vi "get_user_details.vi"(11 "error in (no error)":errorcluster) -> (4 "Name 2":string caption="Enter your name", 6 "Birthday 2":timestamp caption="Select Birthday" format="%<%x>T", 8 "Back_out":T1 caption="Back", 10 "path":path, 15 "error out":errorcluster)   [LabVIEW 2023]
doc: "get the user details."
uses:
  custom_elements/continue.ctl
  custom_elements/back_button.ctl
  <vilib>/Utility/error.llb/Trim Whitespace One-Sided.vi
panel:
  in  "Back":T1
  in  "stop":T2
  in  "Name":string caption="The Name Bestowed Upon Thee"
  in  "Birthday":timestamp caption="The Day of Thy First Light" format="%<%x>T"
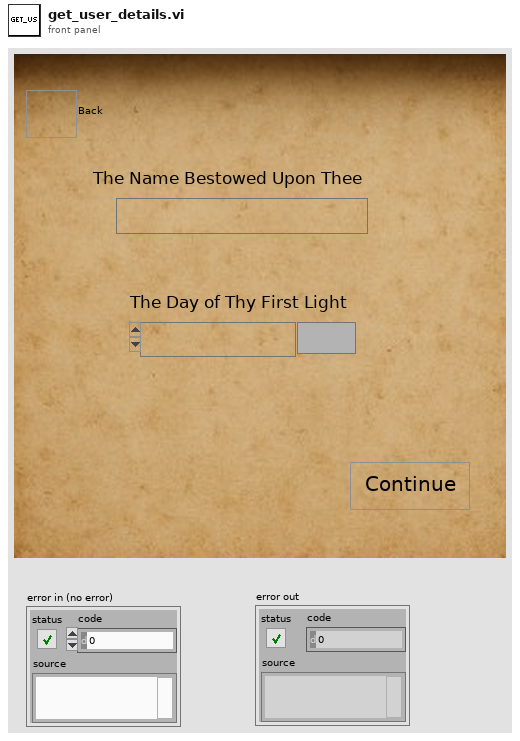
[diagram p1: front panel]
types:
  T1 = typedef "back_button.ctl" = bool
  T2 = typedef "continue.ctl" = bool
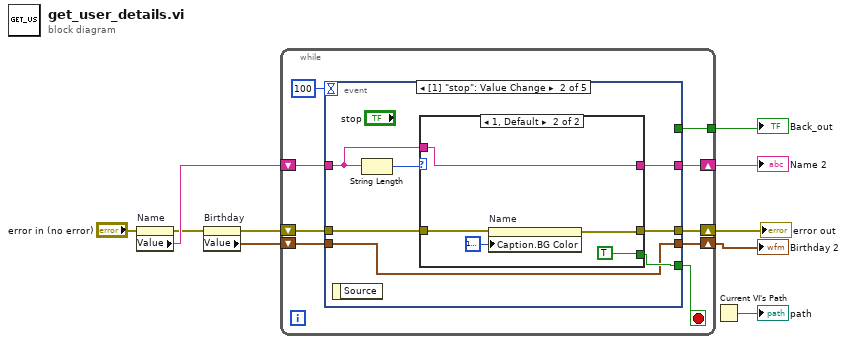
[diagram p0: block diagram]
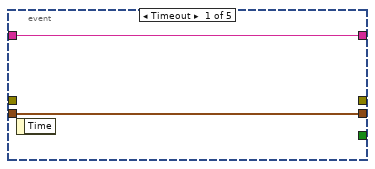
[diagram p2: hidden frame]
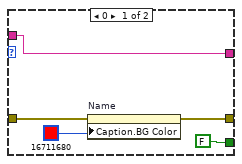
[diagram p3: hidden frame]
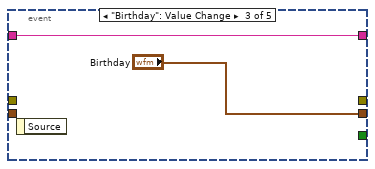
[diagram p4: hidden frame]
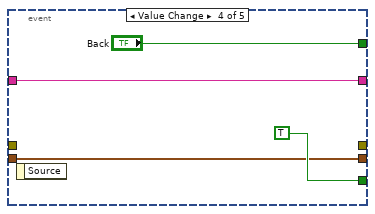
[diagram p5: hidden frame]
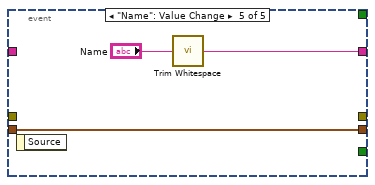
[diagram p6: hidden frame]
diagram:
  n1 = property on="Name" class="Str"(error in="error in (no error)") -> (error out=w3:errorcluster, "Value"=w6:string)  [unwired: 1 in, 1 out]
  n2 = property on="Birthday" class="AbsTime (strict)"(error in=w3) -> (error out=w2:errorcluster, "Value"=w5:timestamp)  [unwired: 1 in, 1 out]
  n3 = while {
    shift-right: [w18] -> w9
    shift-left: w6 -> [w13]
    tunnel: [w15] -> w7
    shift-right: [w17] -> w10
    shift-left: w5 -> [w14]
    shift-right: [w11] -> w1
    shift-left: w2 -> [w12]
    stop <- w16 stop-if-true
    n4 = event shown="[1] \"stop\": Value Change" {
      selector: _ -> [_ _ _ _ _]
      dyn-events: _ -> [_ _ _ _ _]
      timeout: 100 -> [_ _ _ _ _]
      tunnel: [w20 w24 w39 w41 w47] -> w18
      tunnel: [w21 w27 "Birthday" w42 w45] -> w17
      tunnel: [_ w28 _ TRUE _] -> w16
      tunnel: [_ _ _ "Back" _] -> w15
      tunnel: w14 -> [w21 w27 _ w42 w45]
      tunnel: w13 -> [w20 w25 w39 w41 _]
      tunnel: w12 -> [_ w23 _ _ _]
      tunnel: [_ w22 _ _ _] -> w11
      event Timeout {
        n5 = event-data() -> ()  [unwired: 1 in, 1 out]
      }
      event Value Change {
        n6 = event-data() -> ()  [unwired: 1 in, 1 out]
        n7 = String Length(string=w25) -> (length=w26:i32)
        n8 = case shown="1, Default" w26 {
          tunnel: [FALSE TRUE] -> w28
          tunnel: w25 -> [w32 w37]
          tunnel: [w32 w37] -> w24
          tunnel: w23 -> [w30 w35]
          tunnel: [w29 w34] -> w22
          frame 0 {
            n9 = property on="Name" class="Str"(error in=w30, "Caption.BG Color"=u32 16711680 ("Caption.Colors:FG Color")) -> (error out=w29:errorcluster)  [unwired: 1 in, 1 out]
          }
          frame 1, Default {
            n10 = property on="Name" class="Str"(error in=w35, "Caption.BG Color"=u32 16777216 ("Caption.Colors:FG Color")) -> (error out=w34:errorcluster)  [unwired: 1 in, 1 out]
          }
        }
      }
      event "Birthday": Value Change {
        n11 = event-data() -> ()  [unwired: 1 in, 1 out]
      }
      event Value Change {
        n12 = event-data() -> ()  [unwired: 1 in, 1 out]
      }
      event "Name": Value Change {
        n13 = event-data() -> ()  [unwired: 1 in, 1 out]
        n14 = call <vilib>:"Trim Whitespace.vi"("string"="Name") -> ("trimmed string"=w47:string)  [unwired: 1 in]
      }
    }
  }
  "Name 2" <- w9
  "Birthday 2" <- w10
  "Back_out" <- w7
  "error out" <- w1
  n15 = Current VI's Path() -> (path=→"path":path)
